vi "Minimum Compatible Version.vi"(8 "Error in":errorcluster caption="Error in (no error)") -> (0 "Error out":errorcluster, 3 "Min-Compatible Version":T1)   [LabVIEW 2017, in "Communicable State Machine.lvlib"]
uses:
  Communicable State Machine.lvlib
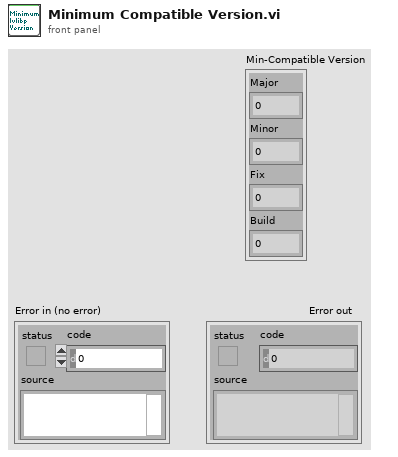
[diagram p1: front panel]
types:
  T1 = cluster{"Major":u16, "Minor":u16, "Fix":u16, "Build":u16}
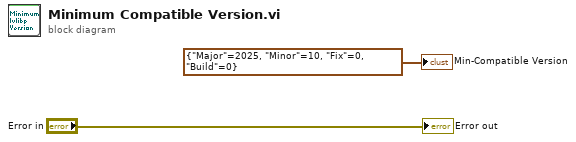
[diagram p0: block diagram]
diagram:
  "Error out" <- "Error in"
  "Min-Compatible Version" <- T1 {"Major"=2025, "Minor"=10, "Fix"=0, "Build"=0} ("Library:Version")
